vi "MC Status.vi"() -> (2 "Subsystem Status":T1)   [LabVIEW 2014]
uses:
  Subsystem Status.ctl
  Global Data.vi
panel:
  in  "Warm Motor Threshold":dbl=90.0
  in  "Warm MC Threshold":dbl=90.0
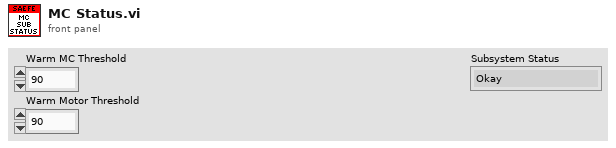
[diagram p1: front panel]
types:
  T1 = typedef "Subsystem Status.ctl" = enum16{"Okay", "Short Warning", "Long Warning", "Return to Pits", "Error", "Danger"}
  T2 = typedef "MC Temp 1.ctl" = cluster{"IGBT A (C)":dbl, "IGBT B (C)":dbl, "IGBT C (C)":dbl, "Gate Driver (C)":dbl}
  T3 = typedef "MC Temp 2.ctl" = cluster{"Control Board (C)":dbl, "RTD #1":dbl, "RTD #2":dbl, "RTD #3":dbl}
  T4 = typedef "MC Temp 3.ctl" = cluster{"RTD #4":dbl, "RTD #5":dbl, "Motor (C)":dbl, "T-Shudder":dbl}
  T5 = typedef "MC Faults.ctl" = cluster{"MC Fault":cluster{"Over-Speed":bool, "Over-Current":bool, "Over-Voltage":bool, "Inverter Over-Temp":bool, "Direction Command":bool, "Inverter Response Time-Out":bool, "Desat Fault":bool, "Hardware Over-Current":bool, "Under-Voltage":bool, "CAN Command Message Lost":bool, "Motor Over-Temp":bool, "Module A Over-Temp":bool, "Module B Over-Temp":bool, "Module C Over-Temp":bool, "PCB Over-Temp":bool, "Gate Driver 1 Over-Temp":bool, "Gate Driver 2 Over-Temp":bool, "Gate Drive 3 Over-Temp":bool, "Current Sensor Fault":bool, "Resolver Not Connected":bool}, "MC Post":u32, "MC RUN":u32}
  T6 = cluster{"Over-Speed":bool, "Over-Current":bool, "Over-Voltage":bool, "Inverter Over-Temp":bool, "Direction Command":bool, "Inverter Response Time-Out":bool, "Desat Fault":bool, "Hardware Over-Current":bool, "Under-Voltage":bool, "CAN Command Message Lost":bool, "Motor Over-Temp":bool, "Module A Over-Temp":bool, "Module B Over-Temp":bool, "Module C Over-Temp":bool, "PCB Over-Temp":bool, "Gate Driver 1 Over-Temp":bool, "Gate Driver 2 Over-Temp":bool, "Gate Drive 3 Over-Temp":bool, "Current Sensor Fault":bool, "Resolver Not Connected":bool}
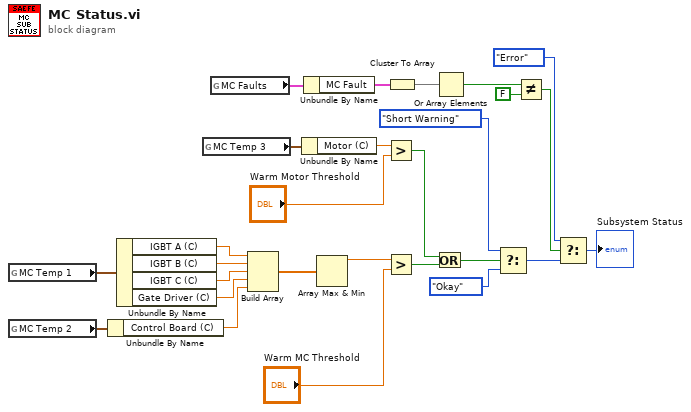
[diagram p0: block diagram]
diagram:
  n1 = global read "Global Data.vi" "MC Temp 1"() -> (w15:T2)
  n2 = global read "Global Data.vi" "MC Temp 2"() -> (w14:T3)
  n3 = Unbundle By Name(w14) -> ("Control Board (C)"=w1:dbl)
  n4 = Unbundle By Name(w15) -> ("IGBT A (C)"=w7:dbl, "IGBT B (C)"=w6:dbl, "IGBT C (C)"=w5:dbl, "Gate Driver (C)"=w4:dbl)
  n5 = global read "Global Data.vi" "MC Temp 3"() -> (w17:T4)
  n6 = global read "Global Data.vi" "MC Faults"() -> (w13:T5)
  n7 = Build Array(w7, w6, w5, w4, w1) -> (w3:dbl[])
  n8 = Unbundle By Name(w17) -> ("Motor (C)"=w16:dbl)
  n9 = Unbundle By Name(w13) -> ("MC Fault"=w11:T6)
  n10 = Array Max & Min(array=w3) -> (max value=w2:dbl)  [unwired: 3 out]
  n11 = Greater?(x=w16, y="Warm Motor Threshold") -> (0:w25:bool)
  n12 = Greater?(x=w2, y="Warm MC Threshold") -> (0:w24:bool)
  n13 = Cluster To Array(cluster=w11) -> (array=w10:bool[])
  n14 = Or(x=w25, y=w24) -> (x .or. y?=w23:bool)
  n15 = Or Array Elements(Boolean array=w10) -> (logical OR=w9:bool)
  n16 = Select(t=Subsystem_Status."Short Warning", s=w23, f=Subsystem_Status."Okay" ("Subsystem Status")) -> (s? t:f=w20:T1)
  n17 = Not Equal?(x=w9, y=FALSE) -> (x != y?=w12:bool)
  n18 = Select(t=Subsystem_Status."Error" ("Subsystem Status"), s=w12, f=w20) -> (s? t:f=→"Subsystem Status":T1)
